vi "Inject.vi"() -> ()   [LabVIEW 2013]
uses:
  Tools/Line.ctl
  Global.vi
panel:
  in  "Inject":bool
  in  "Positions":i32[](array[numeric])
  in  "Injection":T1
  out "#":i32
  in  "SEQs":T1[](array[typedef])
  in  "Save":path
  in  "Stop Button":bool
  in  "Open":path
  in  "Save Button":bool
  in  "Load Button":bool
  # "Inject"
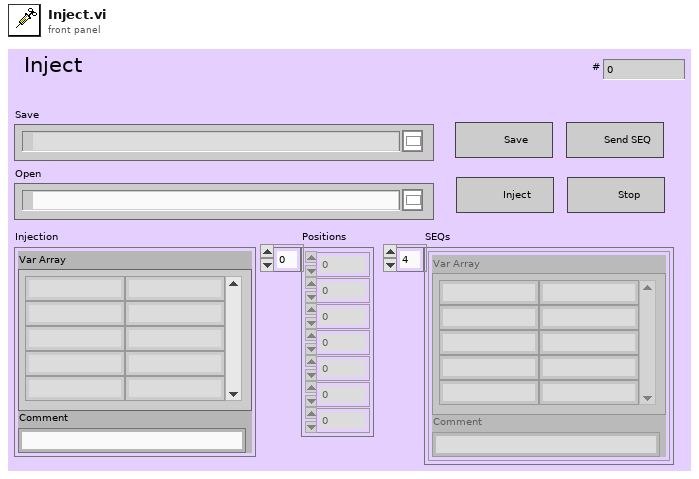
[diagram p1: front panel]
types:
  T1 = typedef "Line.ctl" = cluster{"Var Array":string[][], "Comment":string}
  T2 = enum16{"Left Button", "Center Button", "Right Button", "Window Close"}
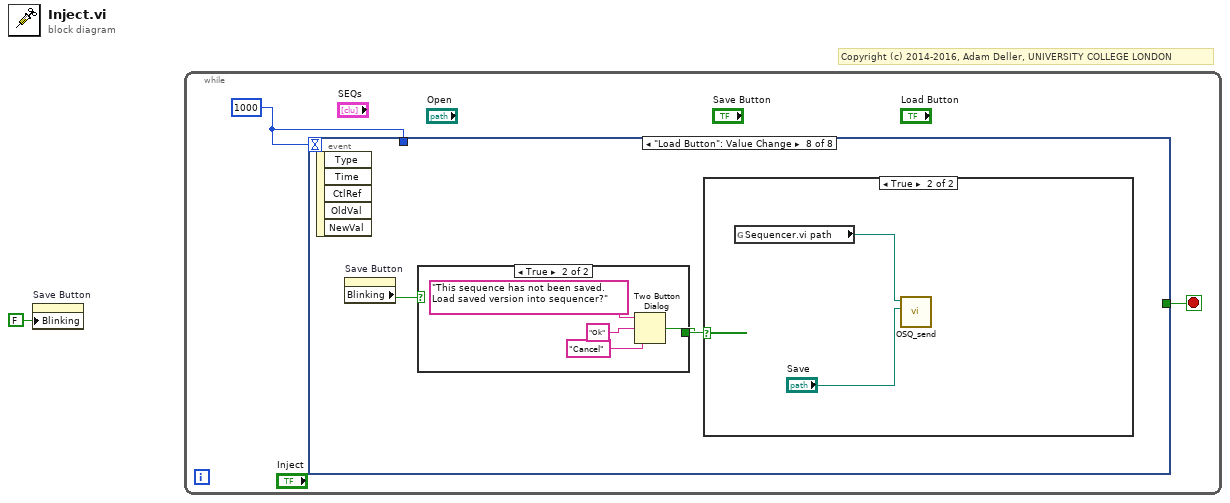
[diagram p0: block diagram]
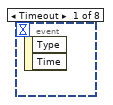
[diagram p2: hidden frame]
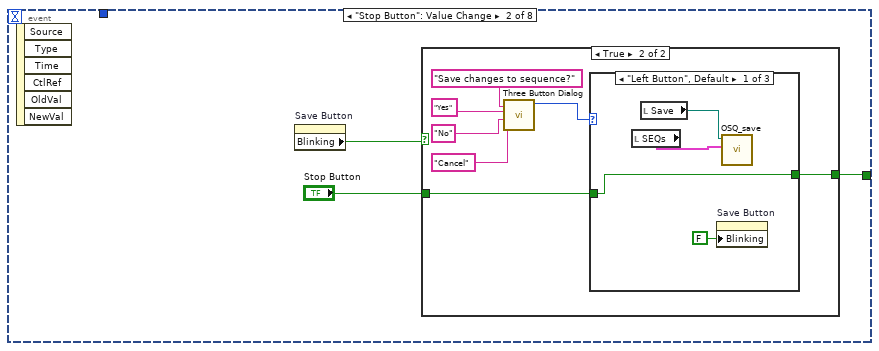
[diagram p3: hidden frame]
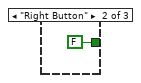
[diagram p5: hidden frame]
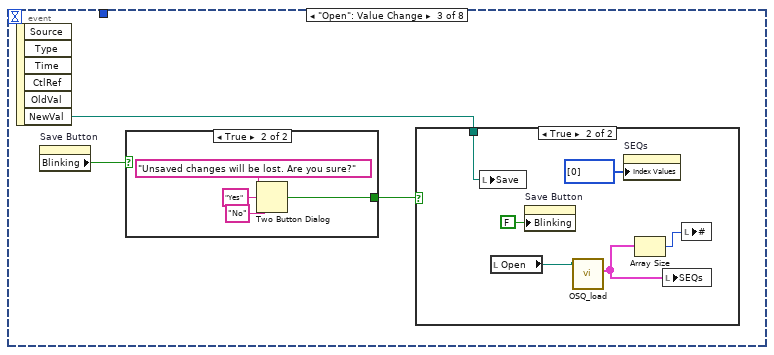
[diagram p7: hidden frame]
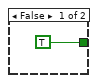
[diagram p9: hidden frame]
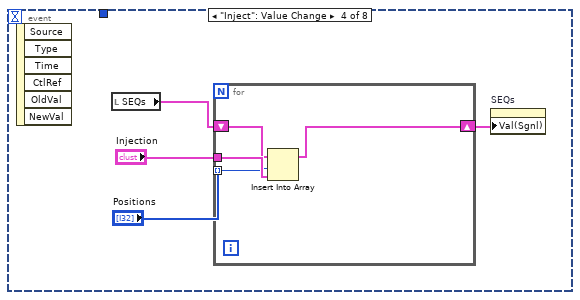
[diagram p10: hidden frame]
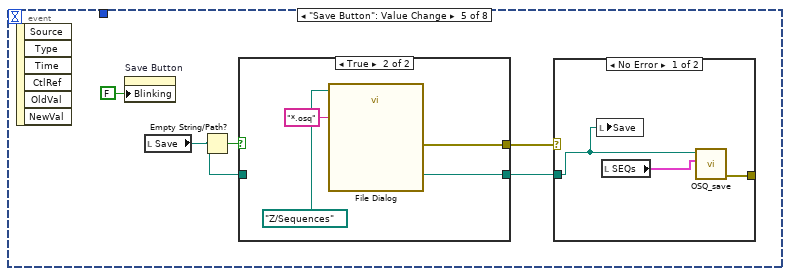
[diagram p11: hidden frame]
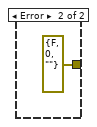
[diagram p12: hidden frame]
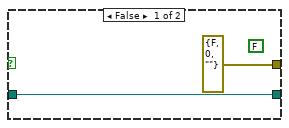
[diagram p13: hidden frame]
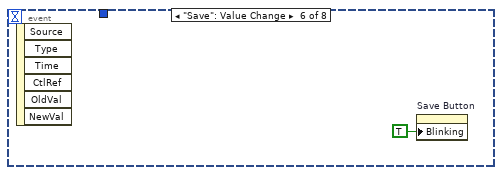
[diagram p14: hidden frame]
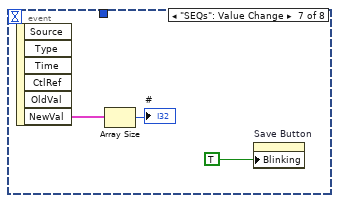
[diagram p15: hidden frame]
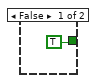
[diagram p17: hidden frame]
diagram:
  # "Copyright (c) 2014-2016, Adam Deller, UNIVERSITY COLLEGE LONDON"
  n1 = property on="Save Button" class="Bool"("Blinking"=FALSE) -> ()  [unwired: 2 in, 2 out]
  n2 = while {
    stop <- w3 stop-if-true
    w2 = 1000
    n3 = event shown="[7] \"Load Button\": Value Change" {
      selector: _ -> [_ _ _ _ _ _ _ _]
      dyn-events: _ -> [_ _ _ _ _ _ _ _]
      timeout: w2 -> [_ _ _ _ _ _ _ _]
      tunnel: [_ w6 _ _ _ _ _ _] -> w3
      tunnel: w2 -> [_ _ _ _ _ _ _ _]
      event Timeout {
        n4 = event-data() -> ()  [unwired: 1 in, 2 out]
      }
      event "Stop Button": Value Change {
        n5 = event-data() -> ()  [unwired: 1 in, 6 out]
        n6 = property on="Save Button" class="Bool"() -> ("Blinking"=w5:bool)  [unwired: 2 in, 2 out]
        n7 = case shown="True" w5 {
          tunnel: [w7 w8] -> w6
          tunnel: "Stop Button" -> [w7 w9]
          frame False {
          }
          frame True {
            n8 = call <vilib>:"Three Button Dialog.vi"("Right Button Text (\"Cancel\")"="Cancel" ("Right Button Text (\"Cancel\")"), "Center Button Text (\"No\")"="No" ("F button name (\"Cancel\")"), "Left Button Text (\"Yes\")"="Yes" ("T button name (\"OK\")"), "message"="Save changes to sequence?") -> ("Which Button?"=w10:T2)  [unwired: 7 in]
            n9 = case shown="\"Left Button\", Default" w10 {
              tunnel: w9 -> [w18 _ w20]
              tunnel: [w18 FALSE ("Stop Button") w20] -> w8
              frame "Left Button", Default {
                n10 = local read "SEQs"() -> (w15:T1[])
                n11 = local read "Save"() -> (w17:path)
                n12 = property on="Save Button" class="Bool"("Blinking"=FALSE) -> ()  [unwired: 2 in, 2 out]
                n13 = call "OSQ_save.vi"("SEQs"=w15, "Save"=w17) -> ()  [unwired: 8 in, 2 out]
              }
              frame "Right Button" {
              }
              frame "Center Button" {
              }
            }
          }
        }
      }
      event "Open": Value Change {
        n14 = event-data() -> ("NewVal"=w21:path)  [unwired: 1 in, 5 out]
        n15 = property on="Save Button" class="Bool"() -> ("Blinking"=w23:bool)  [unwired: 2 in, 2 out]
        n16 = case shown="True" w23 {
          tunnel: [TRUE w31] -> w22
          frame False {
          }
          frame True {
            n17 = Two Button Dialog(message="Unsaved changes will be lost. Are you sure?", 1:"No" ("F button name (\"Cancel\")"), 2:"Yes" ("T button name (\"OK\")")) -> (T button?=w31:bool)
          }
        }
        n18 = case shown="True" w22 {
          tunnel: w21 -> [_ w29]
          frame False {
          }
          frame True {
            n19 = local write "Save"(w29) -> ()
            n20 = local read "Open"() -> (w27:path)
            n21 = property on="Save Button" class="Bool"("Blinking"=FALSE) -> ()  [unwired: 2 in, 2 out]
            n22 = call "OSQ_load.vi"("Open"=w27) -> ("SEQs"=w25:T1[])  [unwired: 7 in, 3 out]
            n23 = property on="SEQs" class="Arr (strict)"("Index Values"=u32[] [0]) -> ()  [unwired: 2 in, 2 out]
            n24 = Array Size(array=w25) -> (size(s)=w24:i32)
            n25 = local write "SEQs"(w25) -> ()
            n26 = local write "#"(w24) -> ()
          }
        }
      }
      event "Inject": Value Change {
        n27 = event-data() -> ()  [unwired: 1 in, 6 out]
        n28 = local read "SEQs"() -> (w36:T1[])
        n29 = for {
          tunnel: "Injection" -> [w42]
          tunnel: "Positions" -> [w41] mode=indexing
          shift-right: [w40] -> w35
          shift-left: w36 -> [w39]
          n30 = Insert Into Array(array=w39, index=w41, new element=w42) -> (w40:T1[])
        }
        n31 = property on="SEQs" class="Arr (strict)"("Val(Sgnl)"=w35) -> ()  [unwired: 2 in, 2 out]
      }
      event "Save Button": Value Change {
        n32 = event-data() -> ()  [unwired: 1 in, 6 out]
        n33 = property on="Save Button" class="Bool"("Blinking"=FALSE) -> ()  [unwired: 2 in, 2 out]
        n34 = local read "Save"() -> (w45:path)
        n35 = Empty String/Path?(string/path=w45) -> (empty?=w46:bool)
        n36 = case shown="True" w46 {
          tunnel: [w53 w57] -> w44
          tunnel: w45 -> [w53 _]
          tunnel: [errorcluster {"status"=FALSE, "code"=0, "source"=""} ("error out") w54] -> w43
          frame False {
            (unwired) FALSE ("cancelled")
          }
          frame True {
            n37 = call "File Dialog"("start path"=path "Z:/Sequences", "pattern (all files)"="*.osq") -> ("selected path"=w57:path, "error out"=w54:errorcluster)  [unwired: 10 in, 2 out]
          }
        }
        n38 = case shown="No Error" w43 {
          tunnel: w44 -> [w49 _]
          tunnel: [w48 errorcluster {"status"=FALSE, "code"=0, "source"=""} ("error out")] -> _
          frame No Error {
            n39 = local write "Save"(w49) -> ()
            n40 = local read "SEQs"() -> (w50:T1[])
            n41 = call "OSQ_save.vi"("SEQs"=w50, "Save"=w49) -> ("error out"=w48:errorcluster)  [unwired: 8 in, 1 out]
          }
          frame Error {
          }
        }
      }
      event "Save": Value Change {
        n42 = event-data() -> ()  [unwired: 1 in, 6 out]
        n43 = property on="Save Button" class="Bool"("Blinking"=TRUE) -> ()  [unwired: 2 in, 2 out]
      }
      event "SEQs": Value Change {
        n44 = event-data() -> ("NewVal"=w60:T1[])  [unwired: 1 in, 5 out]
        n45 = Array Size(array=w60) -> (size(s)=→"#":i32)
        n46 = property on="Save Button" class="Bool"("Blinking"=TRUE) -> ()  [unwired: 2 in, 2 out]
      }
      event "Load Button": Value Change {
        n47 = event-data() -> ()  [unwired: 1 in, 5 out]
        n48 = property on="Save Button" class="Bool"() -> ("Blinking"=w63:bool)  [unwired: 2 in, 2 out]
        n49 = case shown="True" w63 {
          tunnel: [TRUE w67] -> w62
          frame False {
          }
          frame True {
            n50 = Two Button Dialog(message="This sequence has not been saved.  Load saved version into sequencer?", 1:"Cancel" ("F button name (\"Cancel\")"), 2:"Ok" ("T button name (\"OK\")")) -> (T button?=w67:bool)
          }
        }
        n51 = case shown="True" w62 {
          frame False {
          }
          frame True {
            n52 = global read "Global.vi" "Sequencer.vi path"() -> (w65:path)
            n53 = call "OSQ_send.vi"("Sequence File"="Save", "vi path"=w65) -> ()  [unwired: 10 in]
          }
        }
      }
    }
  }
